vi "EMD8216 WDT read.vi"(10 "time":u16, 11 "CardID":u32) -> (0 "enable out":u8, 1 "state":u8[](array[numeric]), 2 "time out":u16, 3 "error_code":u32)   [LabVIEW 2009, in "EMD8216_64.lvlib"]
doc: "EMD8216Status EMD8216_WDT_read(u32 CardID,u16 *time,u8 state[2],u8 *enable);"
uses:
  EMD8216_64.lvlib
  <userlib>/EMD8216_64/EMD8216_64.dll
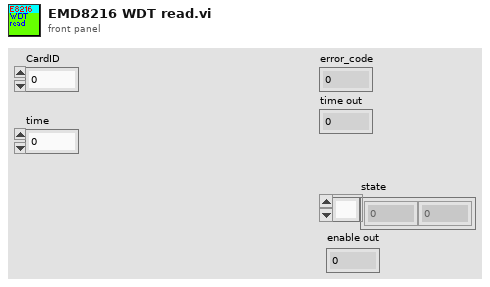
[diagram p1: front panel]
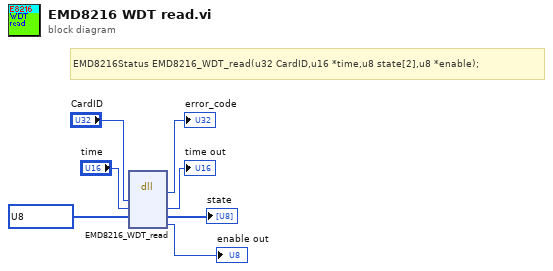
[diagram p0: block diagram]
diagram:
  # "EMD8216Status EMD8216_WDT_read(u32 CardID,u16 *time,u8 state[2],u8 *enable);"
  n1 = dll-call lib="C:/Program Files/National Instruments/LabVIEW 2017/user.lib/EMD8216_64/EMD8216_64.*" fn="EMD8216_WDT_read"("CardID"="CardID", "time"="time", "state"=u8[] ?) -> ("return type"=→"error_code":u32, "time"=→"time out":u16, "state"=→"state":u8[], "enable"=→"enable out":u8)  [unwired: 5 in, 2 out]
